vi "Quick Load Audio File (Polymorphic Template).vi"   [LabVIEW 2020]
uses:
  Private/Result To Error.vi
  dc509e6d-59c1-4a7a-bac3-014c3c6b5a28.vi/48425bba-55d9-4e6a-8c36-a07ede1ba4ab.vi
  ed691427-ca1e-430d-8efd-443bc37f0ad6.vi/48425bba-55d9-4e6a-8c36-a07ede1ba4ab.vi
  <vilib>/Utility/error.llb/Error Cluster From Error Code.vi
  9fc1907d-a31a-455c-b350-5e2e04f7c12e.vi
  8a37d0f7-842a-45b0-a983-25f93089b3b0.vi
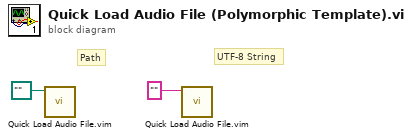
[diagram p0: block diagram]
diagram:
  # "UTF-8 String"
  # "Path"
  n1 = call "Quick Load Audio File.vim"("Path"=path "" ("Path In")) -> ()  [unwired: 5 in, 6 out]
  n2 = call "Quick Load Audio File.vim"("Path"="") -> ()  [unwired: 5 in, 6 out]
